vi "Get SMO Database Paths.vi"(5 "getAll Cluster":variant, 7 "Paths":string="llab_038:d000(TEST_TABLE--Temperature(Kelvin))\nllab_038:d002(TEST_TABLE--voltage 2(volts))\nllab_038:b000(TEST_TABLE--ON?())\nllab_038:v001(TEST_TABLE--sample())", 8 "error in (no error)":errorcluster, 11 "Inst.TC in":refnum<class "Inst.TC.lvclass">) -> (0 "error out":errorcluster, 2 "Paths":string, 3 "Inst.TC out":refnum<class "Inst.TC.lvclass">)   [LabVIEW 2019, in "Inst.TC.lvclass"]
uses:
  Inst.TC.lvclass
  Typedefs/Inst.TC.getAll--Cluster.ctl
  <userlib>/LevyLab/LV-Data/LV-Data.PG/LV-Data.PGSQL.lvclass
  <userlib>/LevyLab/Configuration/Configuration.lvclass
  Typedefs/Inst.TC.DefaultPGSQLPaths--Cluster.ctl
  fb193c0d-8423-4c87-b4cd-4b5ae1b3520d.vi
  <userlib>/LevyLab/Instrument Framework/Instrument/Instrument.lvclass
  <userlib>/LevyLab/Instrument Framework/Instrument Types/Cryostat/Instrument.Cryostat.lvclass
  <userlib>/LevyLab/LV-Data/LV-Data.PG/API/Write Variable (one-row).vi
  C:/Program Files (x86)/National Instruments/LabVIEW 2019/user.lib/LevyLab/Instrument Framework/Instrument/Instrument.lvclass
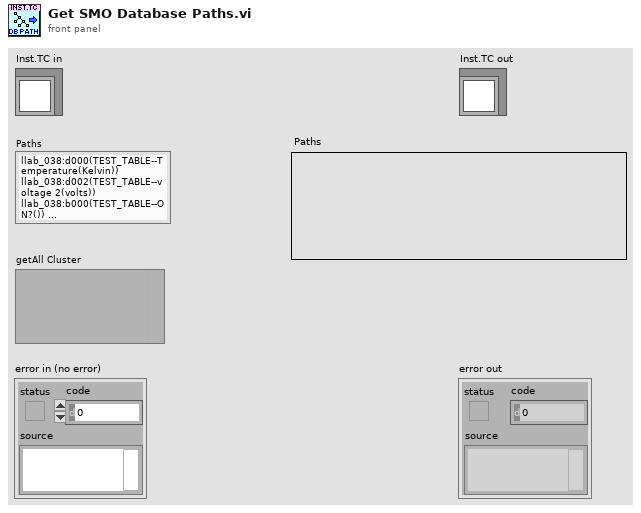
[diagram p1: front panel]
types:
  T1 = typedef "Inst.TC.lvclass/Inst.TC.DefaultPGSQLPaths--Cluster.ctl" = cluster{"CF":string, "CF_Z":string, "MNK":string, "MNK_Z":string}
  T2 = typedef "Inst.TC.lvclass/Inst.TC.getAll--Cluster.ctl" = cluster{"R":dbl[], "T":dbl[], "I":dbl[], "AVS Names":string, "Calibrations":string}
  T3 = typedef "FP-TC-Shared.lvclass/LC Type--Enum.ctl" = enum16{"CF_FP", "CF_TC", "CF_TC_Z", "MNK_FP", "MNK_TC", "MNK_TC_Z", "unknown"}
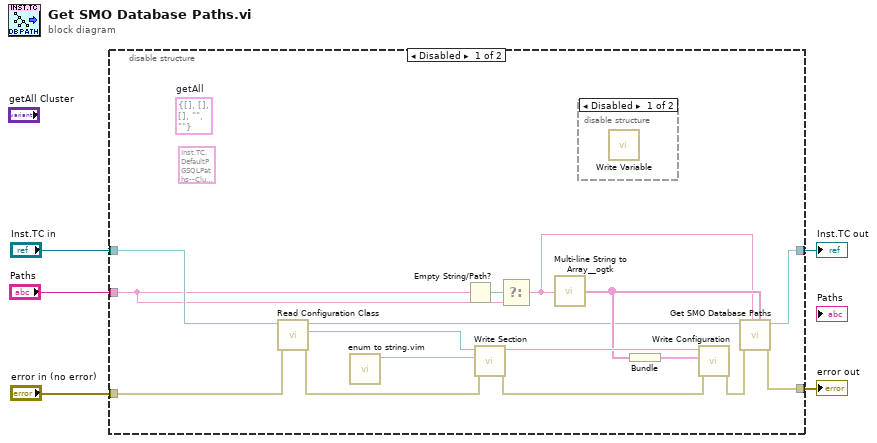
[diagram p0: block diagram]
diagram:
  n1 = disable-structure shown="Disabled" {
    disable-tunnel: [w10 w24] -> w5
    disable-tunnel: "error in (no error)" -> [w9 w24]
    disable-tunnel: [w8 w25] -> w3
    disable-tunnel: "Inst.TC in" -> [w7 w25]
    disable-tunnel: "Paths" -> [w6 _]
    frame Disabled {
      (unwired) T1 {"CF"="llab_015:d001(Leiden CF900--CF_TC_R0(ohms))\nllab_015:d002(Leiden CF900--CF_TC_R1(ohms))\nllab_015:d003(Leiden CF900--CF_TC_R2(ohms))\nllab_015:d004(Leiden CF900--CF_TC_R3(ohms))\nllab_015:d005(Leiden CF900--CF_TC_R4(ohms))\nllab_015:d006(Leiden CF900--CF_TC_R5(ohms))\nllab_015:d007(Leiden CF900--CF_TC_R6(ohms))\nllab_015:d008(Leiden CF900--CF_TC_R7(ohms))\nllab_015:d009(Leiden CF900--CF_TC_T0(mK))\nllab_015:d010(Leiden CF900--CF_TC_T1(mK))\nllab_015:d011(Leiden CF900--CF_TC_T2(mK))\nllab_015:d012(Leiden CF900--CF_TC_T3(mK))\nllab_015:d013(Leiden CF900--CF_TC_T4(mK))\nllab_015:d014(Leiden CF900--CF_TC_T5(mK))\nllab_015:d015(Leiden CF900--CF_TC_T6(mK))\nllab_015:d016(Leiden CF900--CF_TC_T7(mK))\nllab_015:d017(Leiden CF900--CF_TC_I0(Amp))\nllab_015:d018(Leiden CF900--CF_TC_I1(Amp))\nllab_015:d019(Leiden CF900--CF_TC_I2(Amp))\nllab_015:d020(Leiden CF900--CF_TC_I3(Amp))\nllab_015:v000(Leiden CF900--CF_TC_description())\nllab_015:v001(Leiden CF900--CF_TC_calibration())", "CF_Z"="llab_015:d021(Leiden CF900--CF_TC_Z_R0(ohms))\nllab_015:d022(Leiden CF900--CF_TC_Z_R1(ohms))\nllab_015:d023(Leiden CF900--CF_TC_Z_R2(ohms))\nllab_015:d024(Leiden CF900--CF_TC_Z_R3(ohms))\nllab_015:d025(Leiden CF900--CF_TC_Z_R4(ohms))\nllab_015:d026(Leiden CF900--CF_TC_Z_R5(ohms))\nllab_015:d027(Leiden CF900--CF_TC_Z_R6(ohms))\nllab_015:d028(Leiden CF900--CF_TC_Z_R7(ohms))\nllab_015:d029(Leiden CF900--CF_TC_Z_R8(ohms))\nllab_015:d030(Leiden CF900--CF_TC_Z_R9(ohms))\nllab_015:d031(Leiden CF900--CF_TC_Z_T0(mK))\nllab_015:d032(Leiden CF900--CF_TC_Z_T1(mK))\nllab_015:d033(Leiden CF900--CF_TC_Z_T2(mK))\nllab_015:d034(Leiden CF900--CF_TC_Z_T3(mK))\nllab_015:d035(Leiden CF900--CF_TC_Z_T4(mK))\nllab_015:d036(Leiden CF900--CF_TC_Z_T5(mK))\nllab_015:d037(Leiden CF900--CF_TC_Z_T6(mK))\nllab_015:d038(Leiden CF900--CF_TC_Z_T7(mK))\nllab_015:d039(Leiden CF900--CF_TC_Z_T8(mK))\nllab_015:d040(Leiden CF900--CF_TC_Z_T9(mK))\nllab_015:v002(Leiden CF900--CF_TC_Z_description())\nllab_015:v003(Leiden CF900--CF_TC_Z_calibration())", "MNK"="llab_011:d000(Leiden CF FP--CF_FP_P1(mbar))\nllab_011:d001(Leiden CF FP--CF_FP_P2(mbar))\nllab_011:d002(Leiden CF FP--CF_FP_P3(mbar))\nllab_011:d003(Leiden CF FP--CF_FP_P4(mbar))\nllab_011:d004(Leiden CF FP--CF_FP_P5(mbar))\nllab_011:d005(Leiden CF FP--CF_FP_P6(mbar))\nllab_011:d006(Leiden CF FP--CF_FP_P7(mbar))\nllab_011:d007(Leiden CF FP--CF_FP_Flow())\nllab_011:d008(Leiden CF FP--CF_FP_MG0(mbar))\nllab_011:d009(Leiden CF FP--CF_FP_MG1(mbar))\nllab_011:d010(Leiden CF FP--CF_FP_MG2(mbar))\nllab_011:d011(Leiden CF FP--CF_FP_MG3(mbar))\nllab_011:d012(Leiden CF FP--CF_FP_MG4(mbar))\nllab_011:d013(Leiden CF FP--CF_FP_MG5(mbar))\nllab_011:d014(Leiden CF FP--CF_FP_PT_on())\nllab_011:d015(Leiden CF FP--CF_FP_PT_W_in_T(K))\nllab_011:d016(Leiden CF FP--CF_FP_PT_W_out_T(K))\nllab_011:d017(Leiden CF FP--CF_FP_PT_He_T(K))\nllab_011:d018(Leiden CF FP--CF_FP_PT_oil_T(K))\nllab_011:d019(Leiden CF FP--CF_FP_PT_P_Low(bar))\nllab_011:d020(Leiden CF FP--CF_FP_PT_P_High(bar))\nllab_011:d021(Leiden CF FP--CF_FP_PT_current(A))\nllab_011:d022(Leiden CF FP--CF_FP_state0())\nllab_011:d023(Leiden CF FP--CF_FP_state1())\nllab_011:d024(Leiden CF FP--CF_FP_state2())\nllab_011:v000(Leiden CF FP--CF_FP_STATE())", "MNK_Z"="llab_024:d020(MNK_18T--MNK_TC_R0(ohms))\nllab_024:d039(MNK_18T--MNK_TC_R1(ohms))\nllab_024:d021(MNK_18T--MNK_TC_R2(ohms))\nllab_024:d022(MNK_18T--MNK_TC_R3(ohms))\nllab_024:d037(MNK_18T--MNK_TC_R4(ohms))\nllab_024:d023(MNK_18T--MNK_TC_R5(ohms))\nllab_024:d024(MNK_18T--MNK_TC_R6(ohms))\nllab_024:d025(MNK_18T--MNK_TC_R7(ohms))\nllab_024:d026(MNK_18T--MNK_TC_T0(mK))\nllab_024:d027(MNK_18T--MNK_TC_T1(mK))\nllab_024:d028(MNK_18T--MNK_TC_T2(mK))\nllab_024:d029(MNK_18T--MNK_TC_T3(mK))\nllab_024:d030(MNK_18T--MNK_TC_T4(mK))\nllab_024:d038(MNK_18T--MNK_TC_T5(mK))\nllab_024:d031(MNK_18T--MNK_TC_T6(mK))\nllab_024:d032(MNK_18T--MNK_TC_T7(mK))\nllab_024:d033(MNK_18T--MNK_TC_I0(Amp))\nllab_024:d034(MNK_18T--MNK_TC_I1(Amp))\nllab_024:d035(MNK_18T--MNK_TC_I2(Amp))\nllab_024:d036(MNK_18T--MNK_TC_I3(Amp))\nllab_024:v005(MNK_18T--MNK_TC_description())\nllab_024:v006(MNK_18T--MNK_TC_calibration())"} ("PGSQL Paths")
      (unwired) T2 {"R"=[], "T"=[], "I"=[], "AVS Names"="", "Calibrations"=""}  # getAll
      n2 = call <userlib>:"Read Configuration Class.vi"("error in (no error)"=w9, "Instrument in"=w7) -> ("error out"=w19:errorcluster, "Configuration"=w16:refnum<class "Configuration.lvclass">, "Instrument out"=w18:refnum<class "Inst.TC.lvclass">)  [unwired: 7 in]
      n3 = call "enum to string.vim"() -> ("string out"=w23:string, "enum in"=w15:T3)  [unwired: 9 in, 1 out]
      n4 = Empty String/Path?(string/path=w6) -> (empty?=w13:bool)
      n5 = call <userlib>:"Write Section.vi"("error in (no error)"=w19, "Section"=w23, "Configuration in"=w16) -> ("error out"=w14:errorcluster, "Configuration out"=w22:refnum<class "Configuration.lvclass">)  [unwired: 7 in]
      n6 = Select(s=w13, f=w6) -> (t=w12:string, s? t:f=w11:string)
      n7 = call <userlib>:"Multi-line String to Array__ogtk.vi"("string"=w11) -> ("lines"=w20:string[])
      n8 = disable-structure shown="Disabled" {
        frame Disabled {
          n9 = call-poly <userlib>:"Write Variable.vi"() -> ()  [unwired: 8 in, 4 out]
        }
        frame Enabled {
        }
      }
      n10 = Bundle("lines"=w20) -> (w21:cluster{"lines":string[]})  [unwired: 1 in]
      n11 = call <userlib>:"Write Configuration.vi"("error in (no error)"=w14, "Variant"=w21, "Configuration in"=w22) -> ("error out"=w17:errorcluster)  [unwired: 7 in, 1 out]
      n12 = call-parent "Get SMO Database Paths.vi"("getAll Cluster"=w20, "Default Paths"=w11, "error in (no error)"=w17, "Instrument in"=w18) -> ("error out"=w10:errorcluster, "Instrument out"=w8:refnum<class "Inst.TC.lvclass">)  [unwired: 5 in, 1 out]
    }
    frame Enabled {
    }
  }
  "error out" <- w5
  "Inst.TC out" <- w3
